vi "9219_Data_to_Class.vi"(8 "error in (no error)":errorcluster, 10 "9219 Config":T1 {"Conversion Time" items=["High Speed", "Best 60 Hz Rejection", "Best 50 Hz Rejection", "High Resolution"]; "TCoupleType" items=["J", "K", "T", "E", "R", "S", "N", "B"]; "DegreeRange" items=["Raw units", "Degrees Kelvin", "Degrees Celsius", "Degrees Fahrenheit", "Degrees Rankine"]; "RtdType" items=["TCR3851"=1, "TCR3750"=2, "TCR3916"=3, "TCR3920"=4, "TCR3911"=5, "TCR3928"=6, "Custom"=0]}, 11 "9219 in":refnum<class "9219.lvclass">) -> (0 "error out":errorcluster, 3 "9219 out":refnum<class "9219.lvclass">)   [LabVIEW 2011, in "Modules.lvlib" / "9219.lvclass"]
uses:
  9219.lvclass
  9219 Config.ctl
  9219.lvclass/9219.ctl
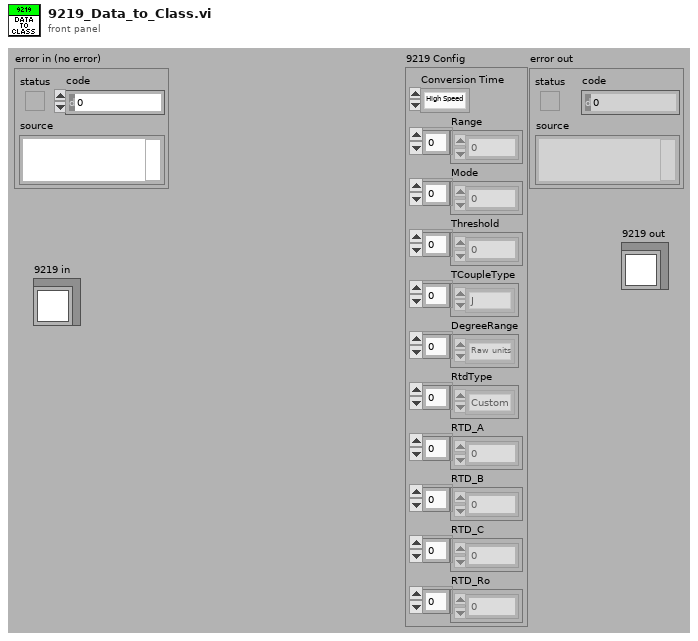
[diagram p1: front panel]
types:
  T1 = typedef "Modules.lvlib/9219.lvclass/9219 Config.ctl" = cluster{"Conversion Time":u16, "Range":u8[], "Mode":u8[], "Threshold":dbl[], "TCoupleType":u8[], "DegreeRange":u8[], "RtdType":u8[], "RTD_A":dbl[], "RTD_B":dbl[], "RTD_C":dbl[], "RTD_Ro":dbl[]}
  T2 = cluster{"Degree range":u32, "Digital threshold":dbl, "Range / Mode":u32, "RTD type":u32, "RTD A":dbl, "RTD B":dbl, "RTD C":dbl, "RTD Ro":dbl, "Thermocouple type":u32}
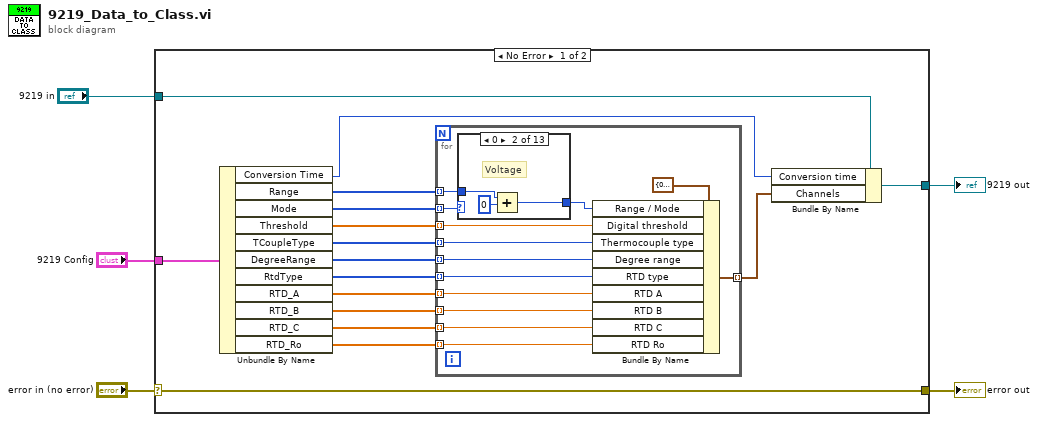
[diagram p0: block diagram]
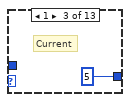
[diagram p3: hidden frame]
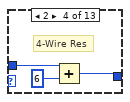
[diagram p4: hidden frame]
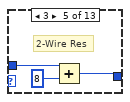
[diagram p5: hidden frame]
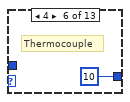
[diagram p6: hidden frame]
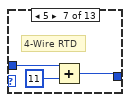
[diagram p7: hidden frame]
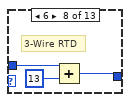
[diagram p8: hidden frame]
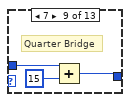
[diagram p9: hidden frame]
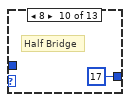
[diagram p10: hidden frame]
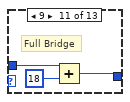
[diagram p11: hidden frame]
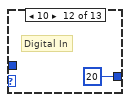
[diagram p12: hidden frame]
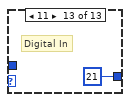
[diagram p13: hidden frame]
diagram:
  n1 = case shown="No Error" "error in (no error)" {
    selector: "error in (no error)" -> [w21 w61]
    tunnel: [w21 w61] -> w4
    tunnel: "9219 Config" -> [w20 _]
    tunnel: [w9 _] -> w2
    tunnel: "9219 in" -> [w6 _]
    frame No Error {
      n2 = Unbundle By Name(w20) -> ("Conversion Time"=w8:u16, "Range"=w19:u8[], "Mode"=w18:u8[], "Threshold"=w17:dbl[], "TCoupleType"=w16:u8[], "DegreeRange"=w15:u8[], "RtdType"=w14:u8[], "RTD_A"=w13:dbl[], "RTD_B"=w12:dbl[], "RTD_C"=w11:dbl[], "RTD_Ro"=w10:dbl[])
      n3 = for {
        tunnel: w19 -> [w23] mode=indexing
        tunnel: w18 -> [w24] mode=indexing
        tunnel: w17 -> [w25] mode=indexing
        tunnel: w16 -> [w26] mode=indexing
        tunnel: w15 -> [w28] mode=indexing
        tunnel: w14 -> [w29] mode=indexing
        tunnel: w13 -> [w30] mode=indexing
        tunnel: w12 -> [w31] mode=indexing
        tunnel: w11 -> [w32] mode=indexing
        tunnel: w10 -> [w33] mode=indexing
        tunnel: [w27] -> w7 mode=indexing
        n4 = case shown="0" w24 {
          tunnel: w23 -> [_ w37 _ w40 w43 _ w47 w50 w53 _ w57 _ _]
          tunnel: [_ w36 u8 5 w39 w42 u8 10 w46 w49 w52 u8 17 w56 u8 20 u8 21] -> w22
          frame Default {
          }
          frame 0 {
            # "Voltage"
            n5 = Add(x=w37, y=u8 0) -> (x+y=w36:u8)
          }
          frame 1 {
            # "Current"
          }
          frame 2 {
            # "4-Wire Res"
            n6 = Add(x=w40, y=u8 6) -> (x+y=w39:u8)
          }
          frame 3 {
            # "2-Wire Res"
            n7 = Add(x=w43, y=u8 8) -> (x+y=w42:u8)
          }
          frame 4 {
            # "Thermocouple"
          }
          frame 5 {
            # "4-Wire RTD"
            n8 = Add(x=w47, y=u8 11) -> (x+y=w46:u8)
          }
          frame 6 {
            # "3-Wire RTD"
            n9 = Add(x=w50, y=u8 13) -> (x+y=w49:u8)
          }
          frame 7 {
            # "Quarter Bridge"
            n10 = Add(x=w53, y=u8 15) -> (x+y=w52:u8)
          }
          frame 8 {
            # "Half Bridge"
          }
          frame 9 {
            # "Full Bridge"
            n11 = Add(x=w57, y=u8 18) -> (x+y=w56:u8)
          }
          frame 10 {
            # "Digital In"
          }
          frame 11 {
            # "Digital In"
          }
        }
        n12 = Bundle By Name(cluster=T2 {"Degree range"=0, "Digital threshold"=0.0, "Range / Mode"=0, "RTD type"=0, "RTD A"=0.0, "RTD B"=0.0, "RTD C"=0.0, "RTD Ro"=0.0, "Thermocouple type"=0} ("Channel"), "Range / Mode"=w22, "Digital threshold"=w25, "Thermocouple type"=w26, "Degree range"=w28, "RTD type"=w29, "RTD A"=w30, "RTD B"=w31, "RTD C"=w32, "RTD Ro"=w33) -> (w27:T2)
      }
      n13 = Bundle By Name(cluster=w6, "Conversion time"=w8, "Channels"=w7) -> (w9:refnum<class "9219.lvclass">)
    }
    frame Error {
    }
  }
  "9219 out" <- w2
  "error out" <- w4
